vi "Update Monitoring Channels.vi"(8 "error in (no error)":errorcluster, 11 "VeriStand DSF in":refnum<class "VeriStand DSF.lvclass">=refnum) -> (0 "error out":errorcluster, 3 "VeriStand DSF out":refnum<class "VeriStand DSF.lvclass">)   [LabVIEW 2019, in "DSF Engine.lvlib" / "VeriStand DSF.lvclass"]
uses:
  VeriStand DSF.lvclass
  DSF Core.lvlibp/Classes/Buffer/Write Buffer 1D DBL.vi
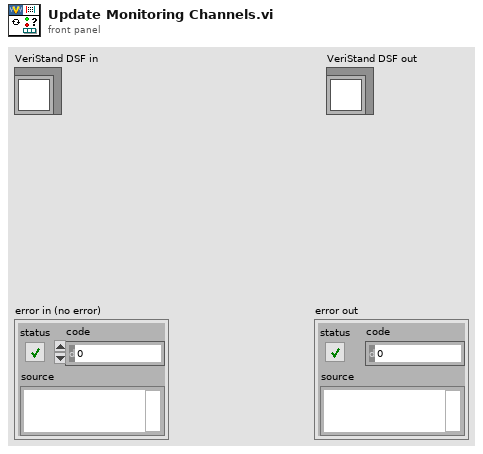
[diagram p1: front panel]
types:
  T1 = typedef "DSF Core.lvlibp/Status Pointer.lvclass/Status Data.ctl" = cluster{"duration":u64, "period":u64, "iteration":u64, "late count":u64}
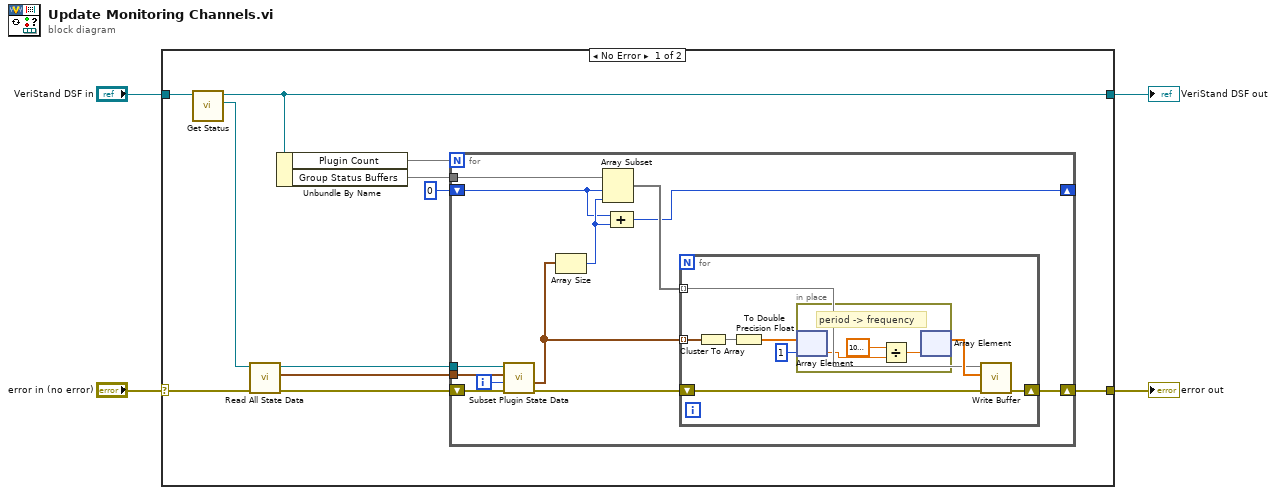
[diagram p0: block diagram]
diagram:
  n1 = case shown="No Error" "error in (no error)" {
    selector: "error in (no error)" -> [w13 w40]
    tunnel: [w7 w40] -> w3
    tunnel: "VeriStand DSF in" -> [w14 w39]
    tunnel: [w15 w39] -> w1
    frame No Error {
      n2 = call "Get Status.vi"("Framework in"=w14) -> ("Status"=w12:refnum<class "Framework Status.lvclass">, "Framework out"=w15:refnum<class "VeriStand DSF.lvclass">)  [unwired: 9 in]
      n3 = call "Read All State Data.vi"("error in (no error)"=w13, "Framework Status in"=w12) -> ("error out"=w11:errorcluster, "all state data"=w9:T1[], "Framework Status out"=w10:refnum<class "Framework Status.lvclass">)  [unwired: 7 in]
      n4 = Unbundle By Name(w15) -> ("Plugin Count"=w8, "Group Status Buffers"=w6)
      n5 = for {
        N: w8 -> [_]
        tunnel: w10 -> [w26]
        tunnel: w9 -> [w25]
        shift-right: [w17] -> w7
        shift-left: w11 -> [w27]
        tunnel: w6 -> [w23]
        shift-right: [w16] -> _
        shift-left: 0 ("index") -> [w20]
        i -> [w24]
        n6 = call "Subset Plugin State Data.vi"("error in (no error)"=w27, "plugin index"=w24, "all state data"=w25, "Framework Status in"=w26) -> ("error out"=w18:errorcluster, "groups state data"=w22:T1[])  [unwired: 4 in, 2 out]
        n7 = Array Size(array=w22) -> (size(s)=w21:i32)
        n8 = Array Subset(array=w23, index=w20, length=w21) -> (w19:void[])
        n9 = Compound Arithmetic op=ADD(w20, w21) -> (w16:i32)
        n10 = for {
          tunnel: w22 -> [w35] mode=indexing
          tunnel: w19 -> [w30] mode=indexing
          shift-right: [w29] -> w17
          shift-left: w18 -> [w28]
          n11 = Cluster To Array(cluster=w35) -> (array=w34:u64[])
          n12 = To Double Precision Float(number=w34) -> (double precision float=w33:dbl[])
          n13 = in-place {
            # "period -> frequency"
            n14 = in-place-array #1(w33, 1) -> (w38:dbl)
            n15 = Divide(x=1000000.0, y=w38) -> (x/y=w36:dbl)
            n16 = in-place-array #1(w36) -> (w31:dbl[])  [unwired: 1 out]
          }
          n17 = call-poly "Write Buffer.vi"("error in (no error)"=w28, "src array in"=w31, "Buffer in"=w30) -> ("error out"=w29:errorcluster)  [unwired: 5 in, 3 out]
        }
      }
    }
    frame Error {
    }
  }
  "error out" <- w3
  "VeriStand DSF out" <- w1
